vi "RSZVB Query Direct Fixture Compensation.vi"(8 "error in (no error)":errorcluster {"code" format="%.0x"}, 9 "Port (1)":i32=1, 10 "Channel (1)":i32=1, 11 "VISA session":refnum<visa-resource-name>) -> (0 "error out":errorcluster {"code" format="%.0x"}, 1 "Direct Fixture Compensation":bool, 3 "dup VISA session":refnum<visa-resource-name>)   [LabVIEW 2011]
doc: "Returns whether a direct fixture compensation has been carried out at port no. <port_no>. A direct fixture compensation resets the offset parameters to zero, the analyzer uses calculated transmission factors instead.\n\nRemote-control command(s):\n[SENSe<Ch>:]CORRection:OFFSet<port_no>:DFComp[:STATe]?"
uses:
  _utility/RSZVB Global Data.vi
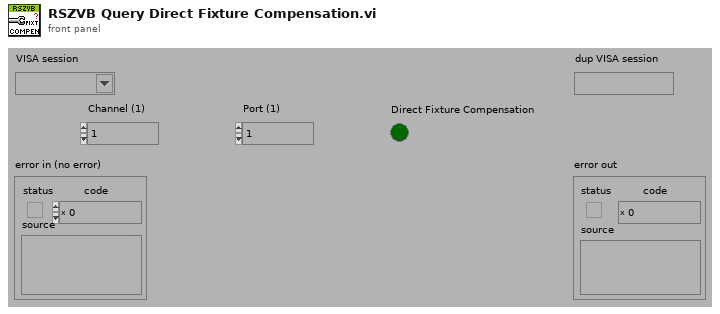
[diagram p1: front panel]
types:
  T1 = cluster{"Error Checking (T: On)":bool, "Installed Options":string[], "Data Valid?":bool, "Ports":i32, "Model":string[], "Option Checking (T: On)":bool}[]
  T2 = cluster{"Error Checking (T: On)":bool, "Installed Options":string[], "Data Valid?":bool, "Ports":i32, "Model":string[], "Option Checking (T: On)":bool}
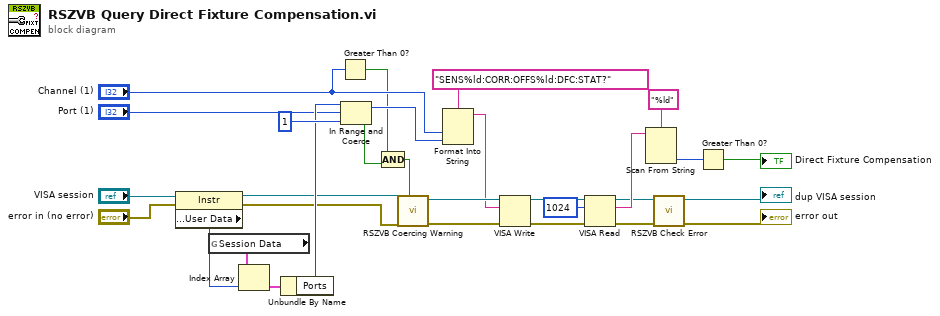
[diagram p0: block diagram]
diagram:
  n1 = property class="Instr"(reference="VISA session", error in="error in (no error)") -> (reference out=w20:refnum<visa-resource-name>, error out=w19:errorcluster, "General Settings:User Data"=w28:u32)
  n2 = global read "RSZVB Global Data.vi" "Session Data"() -> (w29:T1)
  n3 = Index Array(array=w29, index=w28) -> (element=w30:T2)
  n4 = Unbundle By Name(w30) -> ("Ports"=w24:i32)
  n5 = Greater Than 0?(x="Channel (1)") -> (x > 0?=w16:bool)
  n6 = In Range and Coerce(upper limit=w24, x="Port (1)", lower limit=1) -> (coerced(x)=w21:i32, In Range?=w18:bool)
  n7 = Compound Arithmetic op=AND(w16, w18) -> (w1:bool)
  n8 = call "RSZVB Coercing Warning.vi"("In Range?"=w1, "error in (no error)"=w19, "VISA session"=w20) -> ("error out"=w15:errorcluster, "dup VISA session"=w14:refnum<visa-resource-name>)  [unwired: 7 in]
  n9 = Format Into String(format string="SENS%ld:CORR:OFFS%ld:DFC:STAT?", "Channel (1)", w21) -> (resulting string=w13:string)  [unwired: 2 in, 1 out]
  n10 = VISA Write(VISA resource name=w14, write buffer=w13, error in (no error)=w15) -> (VISA resource name out=w12:refnum<visa-resource-name>, error out=w11:errorcluster)  [unwired: 1 out]
  n11 = VISA Read(VISA resource name=w12, byte count=u32 1024, error in (no error)=w11) -> (VISA resource name out=w4:refnum<visa-resource-name>, read buffer=w8:string, error out=w5:errorcluster)  [unwired: 1 out]
  n12 = Scan From String(format string="%ld", input string=w8) -> (output 1=w7:i32)  [unwired: 3 in, 3 out]
  n13 = call "RSZVB Check Error.vi"("error in (no error)"=w5, "VISA session"=w4) -> ("error out"=→"error out":errorcluster, "dup VISA session"=→"dup VISA session":refnum<visa-resource-name>)  [unwired: 8 in]
  n14 = Greater Than 0?(x=w7) -> (x > 0?=→"Direct Fixture Compensation":bool)
